vi "Add Error Template Core.vi"(8 "error in (no error)":errorcluster, 10 "String to Append":string, 11 "Error":enum16{"User Defined Error"}(ring)) -> (0 "error out":errorcluster)   [LabVIEW 2021, in "Errors_CIF_U.lvlib"]
doc: "This reentrant VI contains the error messages. It is called by a wrapper that is inlined for optimal performance. This VI is not inlined to minimize memory impact."
uses:
  Errors_CIF_U.lvlib
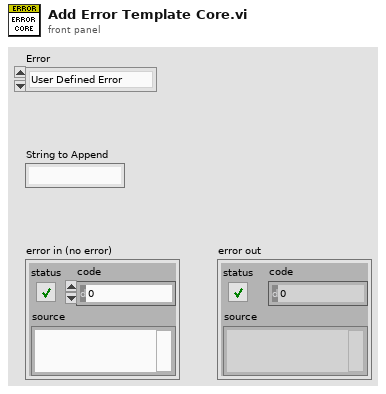
[diagram p1: front panel]
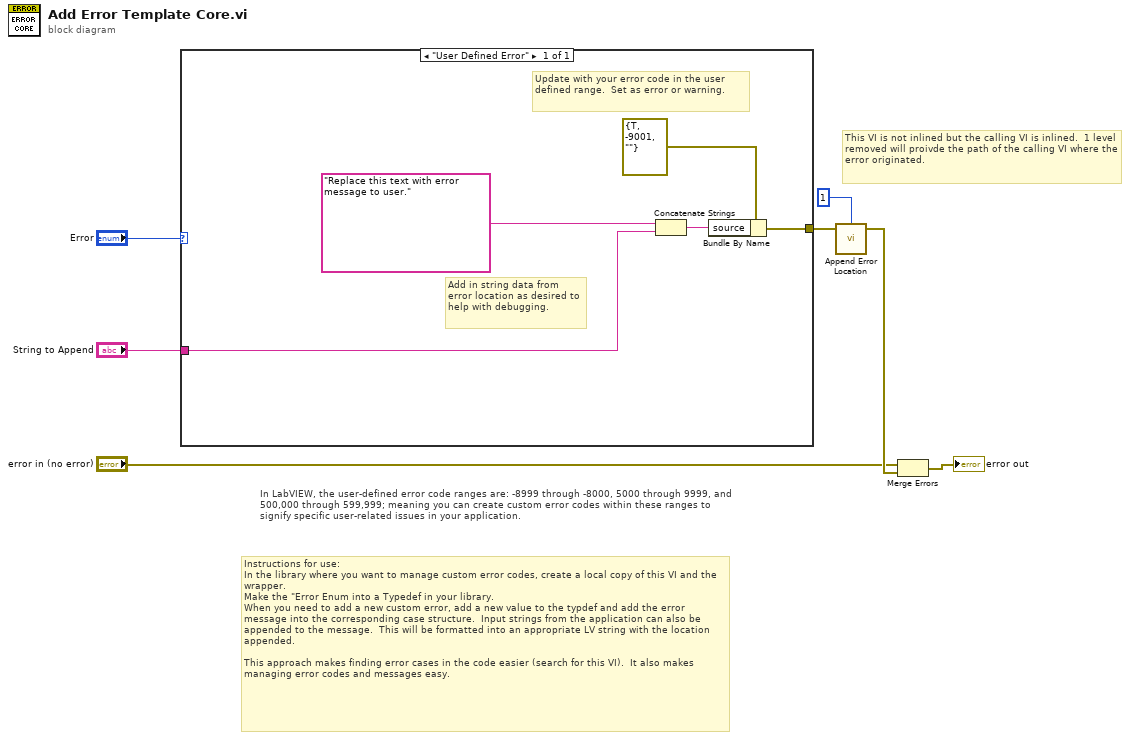
[diagram p0: block diagram]
diagram:
  # "This VI is not inlined but the calling VI is inlined.  1 level removed will proivde the path of the calling VI where the error originated."
  # "Instructions for use:\nIn the library where you want to manage custom error codes, create a local copy of this VI and the wrapper.\nMake the \"Error Enum into a Typedef in your library.\nWhen you need to add a new custom error, add a new value to the typdef and add the error message into the corresponding case structure.  Input strings from the application can also be appended to the message.  This will be formatted into an appropriate LV string with the location appended.  \n\nThis approach makes finding error cases in the code easier (search for this VI).  It also makes managing error codes and messages easy."
  # "In LabVIEW, the user-defined error code ranges are: -8999 through -8000, 5000 through 9999, and 500,000 through 599,999; meaning you can create custom error codes within these ranges to signify specific user-related issues in your application."
  n1 = case shown="\"User Defined Error\"" "Error" {
    tunnel: "String to Append" -> [w9]
    tunnel: [w11] -> w6
    frame "User Defined Error" {
      # "Add in string data from error location as desired to help with debugging."
      # "Update with your error code in the user defined range.  Set as error or warning."
      n2 = Concatenate Strings("Replace this text with error message to user." ("source"), w9) -> (w8:string)
      n3 = Bundle By Name(cluster=errorcluster {"status"=TRUE, "code"=-9001, "source"=""} ("Invalid ID"), "source"=w8) -> (w11:errorcluster)
    }
  }
  n4 = call "Append Error Location.vi"("error in (no error)"=w6, "Chain Depth"=1) -> ("error out"=w7:errorcluster)  [unwired: 3 in]
  n5 = Merge Errors("error in (no error)", w7) -> (→"error out":errorcluster)
